vi "PlotReleaseByYear.vi"() -> ()   [LabVIEW 2024]
uses:
  CV_Shared_Library/CV_Shared_Library.lvlib
panel:
  out "Array":string[][](array[string])
  in  "map 2":map{i32, cluster{"total":i32, "store date":i32}}(c390)={1935={"total"=4, "store date"=4}, 1936={"total"=19, "store date"=19}, 1937={"total"=34, "store date"=33}, 1938={"total"=44, "store date"=44}, 1939={"total"=80, "store date"=79}, 1940={"total"=111, "store date"=111}, 1941={"total"=154, "store date"=151}, 1942={"total"=192, "store date"=188}, 1943={"total"=190, "store date"=185}, 1944={"total"=190, "store date"=187}, 1945={"total"=198, "store date"=185}, 1946={"total"=263, "store date"=218}, 1947={"total"=280, "store date"=216}, 1948={"total"=328, "store date"=227}, 1949={"total"=317, "store date"=197}, 1950={"total"=313, "store date"=71}, 1951={"total"=376, "store date"=58}, 1952={"total"=424, "store date"=58}, 1953={"total"=476, "store date"=51}, 1954={"total"=524, "store date"=62}, 1955={"total"=549, "store date"=28}, 1956={"total"=584, "store date"=31}, 1957={"total"=549, "store date"=13}, 1958={"total"=482, "store date"=22}, 1959={"total"=460, "store date"=28}, 1960={"total"=436, "store date"=29}, 1961={"total"=458, "store date"=36}, 1962={"total"=476, "store date"=36}, 1963={"total"=493, "store date"=32}, 1964={"total"=518, "store date"=34}, 1965={"total"=539, "store date"=46}, 1966={"total"=568, "store date"=90}, 1967={"total"=535, "store date"=96}, 1968={"total"=580, "store date"=33}, 1969={"total"=613, "store date"=76}, 1970={"total"=629, "store date"=45}, 1971={"total"=615, "store date"=36}, 1972={"total"=703, "store date"=49}, 1973={"total"=910, "store date"=48}, 1974={"total"=818, "store date"=30}, 1975={"total"=993, "store date"=42}, 1976={"total"=937, "store date"=52}, 1977={"total"=953, "store date"=101}, 1978={"total"=897, "store date"=107}, 1979={"total"=717, "store date"=114}, 1980={"total"=783, "store date"=96}, 1981={"total"=784, "store date"=71}, 1982={"total"=802, "store date"=115}, 1983={"total"=872, "store date"=100}, 1984={"total"=1021, "store date"=243}, 1985={"total"=1157, "store date"=345}, 1986={"total"=1072, "store date"=202}, 1987={"total"=1172, "store date"=222}, 1988={"total"=1230, "store date"=114}, 1989={"total"=1361, "store date"=55}, 1990={"total"=1313, "store date"=49}, 1991={"total"=1254, "store date"=53}, 1992={"total"=1286, "store date"=59}, 1993={"total"=1382, "store date"=78}, 1994={"total"=1373, "store date"=153}, 1995={"total"=1157, "store date"=121}, 1996={"total"=817, "store date"=55}, 1997={"total"=735, "store date"=62}, 1998={"total"=787, "store date"=90}, 1999={"total"=661, "store date"=58}, 2000={"total"=721, "store date"=55}, 2001={"total"=679, "store date"=82}, 2002={"total"=789, "store date"=88}, 2003={"total"=845, "store date"=316}, 2004={"total"=976, "store date"=577}, 2005={"total"=969, "store date"=443}, 2006={"total"=1019, "store date"=421}, 2007={"total"=1089, "store date"=763}, 2008={"total"=1189, "store date"=943}, 2009={"total"=1371, "store date"=1166}, 2010={"total"=1325, "store date"=1273}, 2011={"total"=1281, "store date"=1211}, 2012={"total"=1027, "store date"=994}, 2013={"total"=990, "store date"=979}, 2014={"total"=1031, "store date"=1028}, 2015={"total"=965, "store date"=965}, 2016={"total"=1189, "store date"=1188}, 2017={"total"=1234, "store date"=1232}, 2018={"total"=1127, "store date"=1127}, 2019={"total"=1237, "store date"=1227}, 2020={"total"=764, "store date"=763}, 2021={"total"=876, "store date"=876}, 2022={"total"=973, "store date"=973}, 2023={"total"=1297, "store date"=1296}, 2024={"total"=1504, "store date"=1495}, 2025={"total"=55, "store date"=54}}
  out "total issues":i32
  out "map":map{i32, cluster{"total":i32, "store date":i32}}(c390)
  out "progress":i32(slide) scale=0.0..68070.0
  in  "Folder Path":path
  # "Export to Spreadsheet to plot it out"
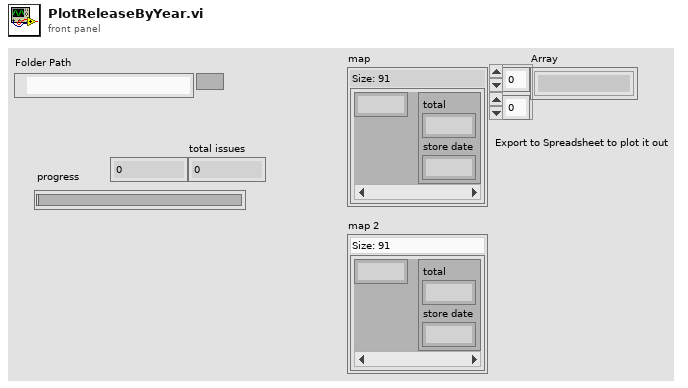
[diagram p1: front panel]
types:
  T1 = typedef "CV_RESTful_Lib.lvlib/local_issue--cluster.ctl" = cluster{"cover_date":timestamp, "id":i32, "cv_id":string, "name":string, "sortable_name":string, "issue_number":string, "deck":string, "description":string, "volume":T2, "store_date":timestamp, "date_last_updated":timestamp, "site_detail_url":string, "cover_url":string, "associated_images":T3[], "characters":T2[], "concepts":T2[], "creators":T4[], "storyArcs":T2[], "teams":T2[], "in collection":bool}
  T2 = typedef "CV_RESTful_Lib.lvlib/cv_issue.generic_credit--cluster.ctl" = cluster{"id":i32, "name":string}
  T3 = typedef "CV_RESTful_Lib.lvlib/cv_issue.associated_image--cluster.ctl" = cluster{"original_url":string, "id":i32}
  T4 = typedef "CV_RESTful_Lib.lvlib/cv_issue.person_credit--cluster.ctl" = cluster{"id":i32, "name":string, "role":string}
  T5 = typedef "LVDateTimeRec.ctl" = cluster{"fractional second":dbl, "second":i32, "minute":i32, "hour":i32, "day of month":i32, "month":i32, "year":i32, "day of week":i32, "day of year":i32, "DST":i32}
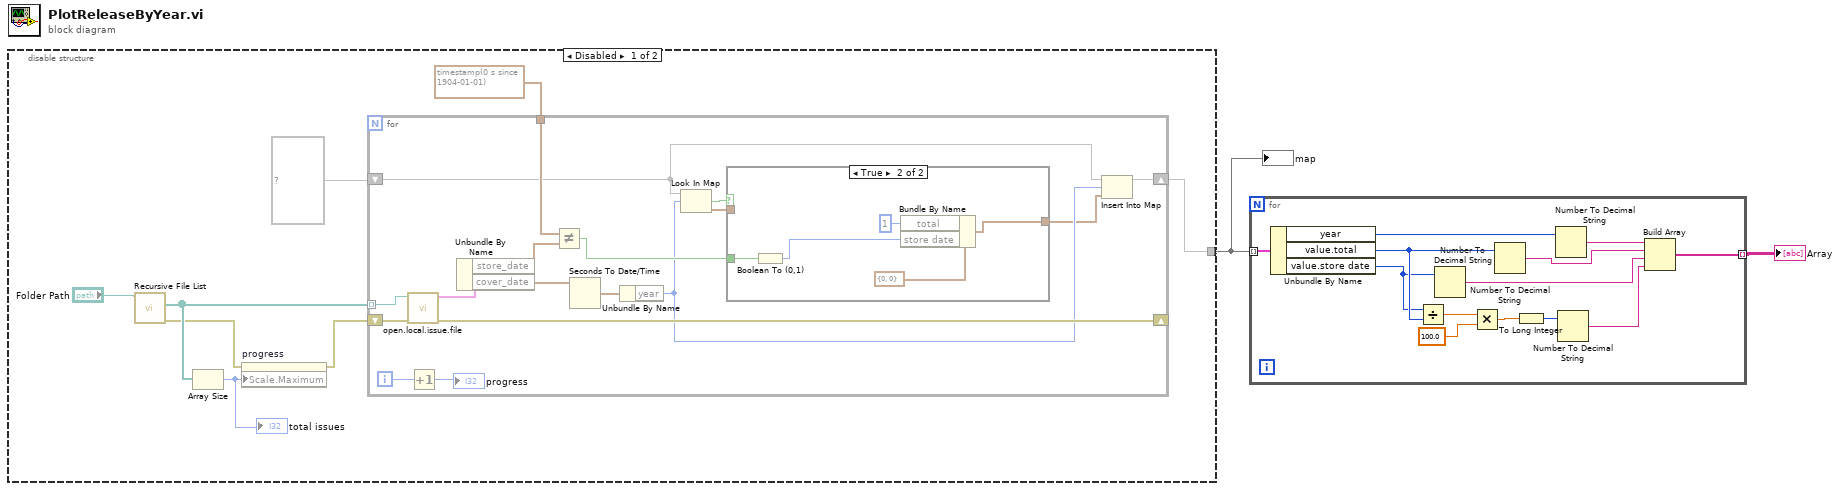
[diagram p0: block diagram]
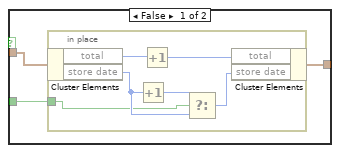
[diagram p2: hidden frame]
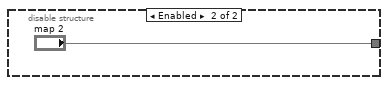
[diagram p3: hidden frame]
diagram:
  n1 = disable-structure shown="Disabled" {
    disable-tunnel: [w4 "map 2"] -> w2
    frame Disabled {
      n2 = call <vilib>:"Recursive File List.vi"("Folder Path"="Folder Path") -> ("error out"=w8:errorcluster, "All Files in Dir"=w9:path[])  [unwired: 6 in, 3 out]
      n3 = Array Size(array=w9) -> (size(s)=w3:i32)
      "total issues" <- w3
      n4 = property on="progress" class="Slide (strict)"(error in=w8, "Scale.Maximum"=w3) -> (error out=w7:errorcluster)  [unwired: 1 in, 1 out]
      n5 = for {
        shift-right: [w23] -> _
        shift-left: w7 -> [w27]
        tunnel: w9 -> [w26] mode=indexing
        tunnel: timestamp(0 s since 1904-01-01) -> [w20]
        shift-right: [w13] -> w4
        shift-left: map{i32, cluster{"total":i32, "store date":i32}} {} ("map") -> [w14]
        i -> [w25]
        n6 = call "open.local.issue.file.vi"("error in (no error)"=w27, "issue json path"=w26) -> ("error out"=w23:errorcluster, "issue"=w22:T1)  [unwired: 8 in]
        n7 = Increment(x=w25) -> (x+1=→"progress":i32)
        n8 = Unbundle By Name(w22) -> ("store_date"=w21:timestamp, "cover_date"=w19:timestamp)
        n9 = Not Equal?(x=w20, y=w21) -> (x != y?=w15:bool)
        n10 = Seconds To Date/Time(time stamp (now)=w19) -> (date time rec=w18:T5)  [unwired: 1 in]
        n11 = Unbundle By Name(w18) -> ("year"=w12:i32)
        n12 = Look In Map(map=w14, key=w12) -> (key not found?=w17:bool, value=w16:cluster{"total":i32, "store date":i32})  [unwired: 1 in]
        n13 = case shown="True" w17 {
          tunnel: w16 -> [w30 _]
          tunnel: w15 -> [w29 w39]
          tunnel: [w28 w37] -> w11
          frame False {
            n14 = in-place {
              in-place-border: w29 -> [w32]
              n15 = in-place-cluster #1(w30) -> ("total"=w36:i32, "store date"=w33:i32)
              n16 = Increment(x=w33) -> (x+1=w34:i32)
              n17 = Increment(x=w36) -> (x+1=w35:i32)
              n18 = Select(t=w34, s=w32, f=w33) -> (s? t:f=w31:i32)
              n19 = in-place-cluster #1("total"=w35, "store date"=w31) -> (w28:cluster{"total":i32, "store date":i32})
            }
          }
          frame True {
            n20 = Boolean To (0,1)(Boolean=w39) -> (0, 1=w38:i16)
            n21 = Bundle By Name(cluster=cluster{"total":i32, "store date":i32} {"total"=0, "store date"=0} ("value"), "total"=1, "store date"=w38) -> (w37:cluster{"total":i32, "store date":i32})
          }
        }
        n22 = Insert Into Map(map in=w14, key=w12, value=w11) -> (map out=w13:map{i32, cluster{"total":i32, "store date":i32}})  [unwired: 2 out]
      }
    }
    frame Enabled {
    }
  }
  "map" <- w2
  n23 = for {
    tunnel: w2 -> [w55] mode=indexing
    tunnel: [w43] -> w1 mode=indexing
    n24 = Unbundle By Name(w55) -> ("year"=w51:i32, "value.total"=w50:i32, "value.store date"=w49:i32)
    n25 = Divide(x=w49, y=w50) -> (x/y=w54:dbl)
    n26 = Number To Decimal String(number=w49) -> (decimal integer string=w45:string)  [unwired: 1 in]
    n27 = Multiply(x=w54, y=100.0) -> (x*y=w52:dbl)
    n28 = Number To Decimal String(number=w50) -> (decimal integer string=w46:string)  [unwired: 1 in]
    n29 = To Long Integer(number=w52) -> (32bit integer=w48:i32)
    n30 = Number To Decimal String(number=w51) -> (decimal integer string=w47:string)  [unwired: 1 in]
    n31 = Number To Decimal String(number=w48) -> (decimal integer string=w44:string)  [unwired: 1 in]
    n32 = Build Array(w47, w46, w45, w44) -> (w43:string[])
  }
  "Array" <- w1
